vi "read_params.vi"(8 "error in (no error)":errorcluster, 11 "NMF in":refnum<class "NMF.lvclass">) -> (0 "error out":errorcluster, 2 "params":T1={"n_components"={"n_components_type"="None", "n_components_int"=0.0}, "init"="None", "solver"="cd", "beta_loss"={"beta_loss_type"="frobenius", "beta_loss_float"=0.0}, "tol"=0.0001, "max_iter"=200.0, "random_state"=0.0, "alpha"=0.0, "l1_ratio"=0.0, "verbose"=0.0, "shuffle"=FALSE, "regularization"="both"}, 3 "NMF out":refnum<class "NMF.lvclass">)   [LabVIEW 2020, in "NMF.lvclass"]
uses:
  NMF.lvclass
  Controls/non_negative_matrix_factorization_params.ctl
  NMF.lvclass/NMF.ctl
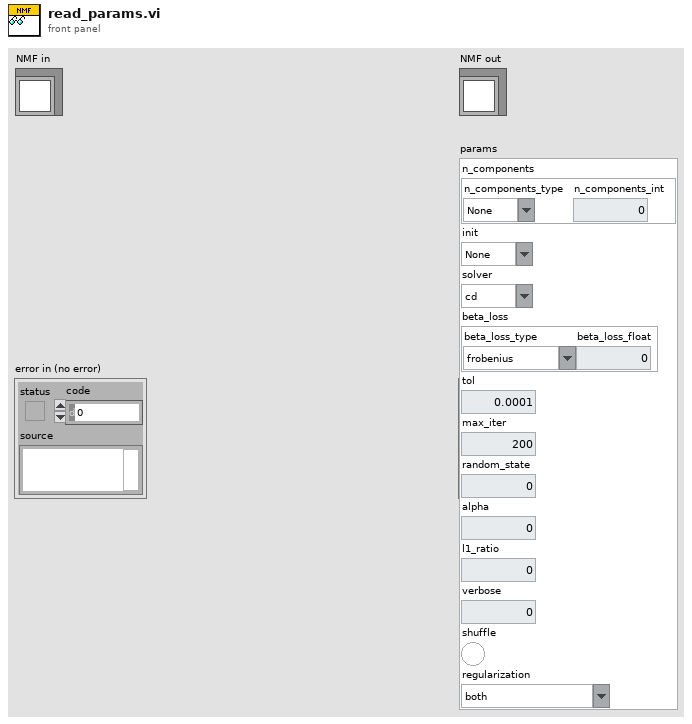
[diagram p1: front panel]
types:
  T1 = typedef "non_negative_matrix_factorization_params.ctl" = cluster{"n_components":cluster{"n_components_type":string, "n_components_int":dbl}, "init":string, "solver":string, "beta_loss":cluster{"beta_loss_type":string, "beta_loss_float":dbl}, "tol":dbl, "max_iter":dbl, "random_state":dbl, "alpha":dbl, "l1_ratio":dbl, "verbose":dbl, "shuffle":bool, "regularization":string}
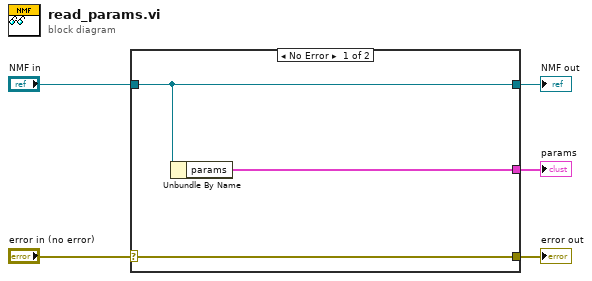
[diagram p0: block diagram]
diagram:
  n1 = case shown="No Error" "error in (no error)" {
    selector: "error in (no error)" -> [w8 w9]
    tunnel: [w8 w9] -> w4
    tunnel: [w7 w10] -> w2
    tunnel: "NMF in" -> [w7 w10]
    tunnel: [w6 _] -> w1
    frame No Error {
      n2 = Unbundle By Name(w7) -> ("params"=w6:T1)
    }
    frame Error {
    }
  }
  "error out" <- w4
  "NMF out" <- w2
  "params" <- w1
